vi "Recieve que bnotifier.vi"() -> ()   [LabVIEW 2022 SP3]
panel:
  out "error out":errorcluster
  in  "stop":bool
  in  "error in (no error)":errorcluster
  out "Get  Que":u8
  out "Get Notifier":u8
  in  "Get Que 1":bool
  in  "Get Nitification":bool
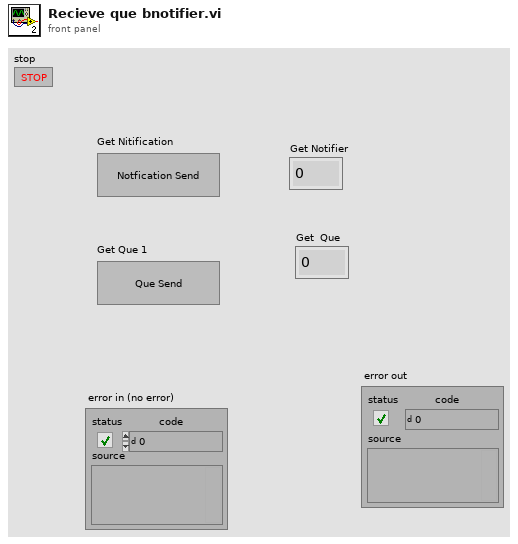
[diagram p1: front panel]
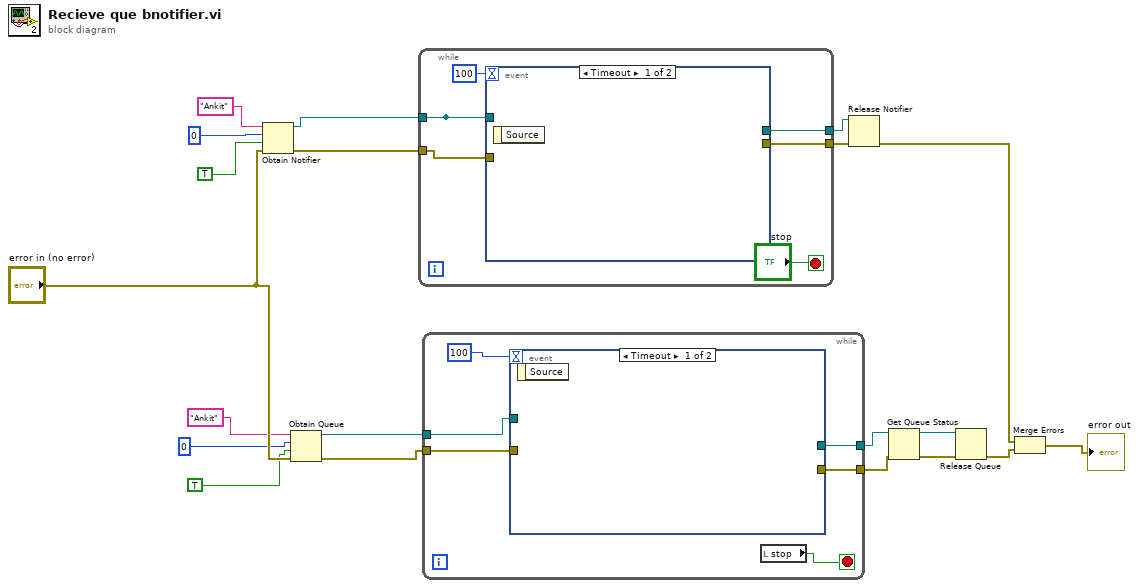
[diagram p0: block diagram]
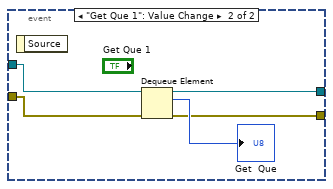
[diagram p2: hidden frame]
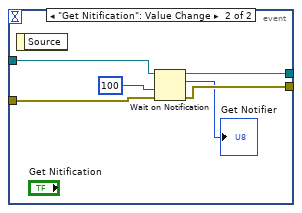
[diagram p3: hidden frame]
diagram:
  n1 = Obtain Notifier(name (unnamed)="Ankit", notification data type=0, create if not found? (T)=TRUE, error in (no error)="error in (no error)") -> (notifier out=w17:refnum<notifier>, error out=w16:errorcluster)  [unwired: 1 out]
  n2 = Obtain Queue(name (unnamed)="Ankit", element data type=0, create if not found? (T)=TRUE, error in (no error)="error in (no error)") -> (queue out=w12:refnum<queue>, error out=w11:errorcluster)  [unwired: 1 in, 1 out]
  n3 = while {
    tunnel: [w24] -> _
    tunnel: w17 -> [w24]
    tunnel: w16 -> [w25]
    tunnel: [w23] -> w15
    tunnel: [w22] -> w14
    stop <- "stop" stop-if-true
    n4 = event shown="[0] Timeout" {
      selector: _ -> [_ _]
      dyn-events: _ -> [_ _]
      timeout: 100 -> [_ _]
      tunnel: w25 -> [_ w31]
      tunnel: w24 -> [_ w30]
      tunnel: [_ w29] -> w23
      tunnel: [_ w28] -> w22
      event Timeout {
        n5 = event-data() -> ()  [unwired: 1 in, 1 out]
      }
      event "Get Nitification": Value Change {
        n6 = event-data() -> ()  [unwired: 1 in, 1 out]
        n7 = Wait on Notification(notifier=w30, timeout in ms (-1)=100, error in (no error)=w31) -> (notifier out=w29:refnum<notifier>, notification=→"Get Notifier":i32, error out=w28:errorcluster)  [unwired: 1 in, 1 out]
      }
    }
  }
  n8 = while {
    tunnel: w12 -> [w36]
    tunnel: w11 -> [w35]
    tunnel: [w34] -> w7
    tunnel: [w33] -> w6
    stop <- w38 stop-if-true
    n9 = event shown="[0] Timeout" {
      selector: _ -> [_ _]
      dyn-events: _ -> [_ _]
      timeout: 100 -> [_ _]
      tunnel: w36 -> [_ w43]
      tunnel: w35 -> [_ w42]
      tunnel: [_ w40] -> w34
      tunnel: [_ w39] -> w33
      event Timeout {
        n10 = event-data() -> ()  [unwired: 1 in, 1 out]
      }
      event "Get Que 1": Value Change {
        n11 = event-data() -> ()  [unwired: 1 in, 1 out]
        n12 = Dequeue Element(queue=w43, error in (no error)=w42) -> (queue out=w40:refnum<queue>, element=→"Get  Que":i32, error out=w39:errorcluster)  [unwired: 1 in, 1 out]
      }
    }
    n13 = local read "stop"() -> (w38:bool)
  }
  n14 = Release Notifier(notifier=w15, error in (no error)=w14) -> (error out=w2:errorcluster)  [unwired: 1 in, 2 out]
  n15 = Get Queue Status(queue=w7, error in (no error)=w6) -> (queue out=w5:refnum<queue>, error out=w4:errorcluster)  [unwired: 1 in, 6 out]
  n16 = Release Queue(queue=w5, error in (no error)=w4) -> (error out=w3:errorcluster)  [unwired: 1 in, 2 out]
  n17 = Merge Errors(w2, w3) -> (→"error out":errorcluster)
